vi "joystick.vi"() -> ()   [LabVIEW 2013]
uses:
  <vilib>/LabVIEW Interface for Arduino/LabVIEW Interface for Arduino.lvlib
panel:
  out "Y":dbl
  out "X":dbl
  in  "stop":bool
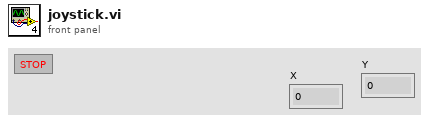
[diagram p1: front panel]
types:
  T1 = typedef "LabVIEW Interface for Arduino.lvlib/Arduino Resource.ctl" = cluster{"VISA resource":refnum<visa-resource-name>, "Board Type":T2, "Connection Type":enum8{"USB / Serial"}, "Bytes Per Packet (15)":u8}
  T2 = typedef "LabVIEW Interface for Arduino.lvlib/Board Type.ctl" = enum16{"Uno", "Dimuelanove w/Atmega 328", "Mega 2560"}
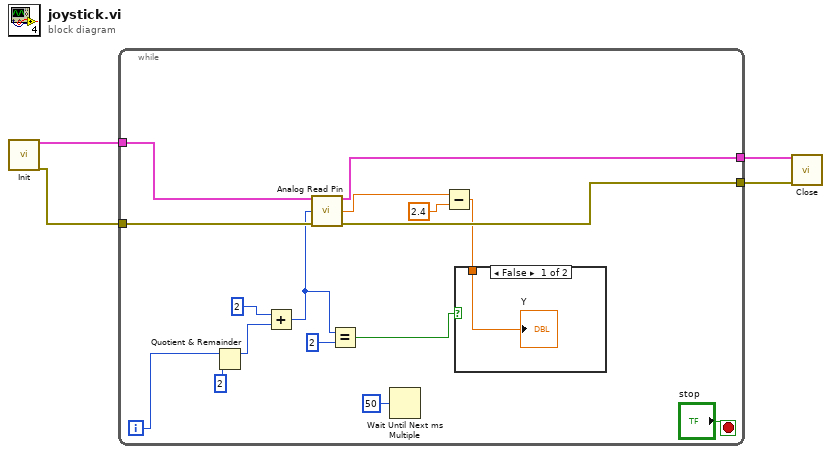
[diagram p0: block diagram]
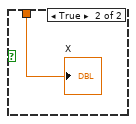
[diagram p2: hidden frame]
diagram:
  n1 = call <vilib>:"Init.vi"() -> ("Arduino Resource"=w3:T1, "error out"=w4:errorcluster)  [unwired: 18 in]
  n2 = while {
    tunnel: w4 -> [w15]
    tunnel: w3 -> [w14]
    tunnel: [w13] -> w2
    tunnel: [w12] -> w1
    i -> [w19]
    stop <- "stop" stop-if-true
    n3 = Quotient & Remainder(x=w19, y=2) -> (x-y*floor(x/y)=w17:i32)  [unwired: 1 out]
    n4 = Add(x=2, y=w17) -> (x+y=w11:i32)
    n5 = call <vilib>:"Analog Read Pin.vi"("Arduino Resource"=w14, "Analog Input Pin (0)"=w11, "error in"=w15) -> ("Arduino Resource"=w13:T1, "Voltage"=w7:dbl, "error out"=w12:errorcluster)  [unwired: 10 in]
    n6 = Equal?(x=w11, y=2) -> (x = y?=w9:bool)
    n7 = Wait Until Next ms Multiple(millisecond multiple=u32 50) -> ()  [unwired: 1 out]
    n8 = Subtract(x=w7, y=2.4) -> (x-y=w6:dbl)
    n9 = case shown="False" w9 {
      tunnel: w6 -> [w21 w22]
      frame False {
        "Y" <- w21
      }
      frame True {
        "X" <- w22
      }
    }
  }
  n10 = call <vilib>:"Close.vi"("Arduino Resource"=w2, "error in"=w1) -> ()  [unwired: 13 in, 1 out]
